vi "SHAPE_GA_Insert Into Population.vi"(6 "Parameters":T3={"Population size"=100, "Generations no."=500, "Significant digits"=4, "Crossover probabality"=0.85, "Mutation mode"=enum."one-point, fixed rate", "Use Gray code?"=FALSE, "Mutation rate"=0.05, "Min mutation rate"=0.0005, "Max mutation rate"=0.25, "Reproduction plan"=enum."Steady-state-replace-worst", "Elitism"=FALSE, "Fmax"=1} {"Max mutation rate" min=0.0 max=1.0; "Min mutation rate" min=0.0 max=1.0; "Mutation rate" min=0.0 max=1.0; "Crossover probabality" min=0.0 max=1.0; "Significant digits" min=1; "Generations no." min=1; "Population size" min=1}, 7 "Fitness Function":T2, 8 "Offsprings":i32[][](array[numeric]), 11 "Population in":T1) -> (3 "Population out":T1)   [LabVIEW 2016, in "Shapelets Search (GA).lvlib"]
doc: "Вставить потомков в популяцию с учетом стратегии замещения особей (reproduction plan)"
uses:
  Shapelets Search (GA).lvlib
  5. Features Optimization/_Optimal Frequency Bands Search/GA_core/GA_tParameters.ctl
  5. Features Optimization/_Optimal Frequency Bands Search/GA_core/GA_tFitness Function.ctl
  5. Features Optimization/_Optimal Frequency Bands Search/GA_core/GA_tPopulation.ctl
  5. Features Optimization/_Optimal Frequency Bands Search/GA_core/GeneticAlgorithm.lvlib
panel:
  # "This VI is a part of BCI Design library, http://www.ru-bci.org \nCopyright © 2020, Sotnikov Peter, All rights reserved. License: GNU GPLv3"
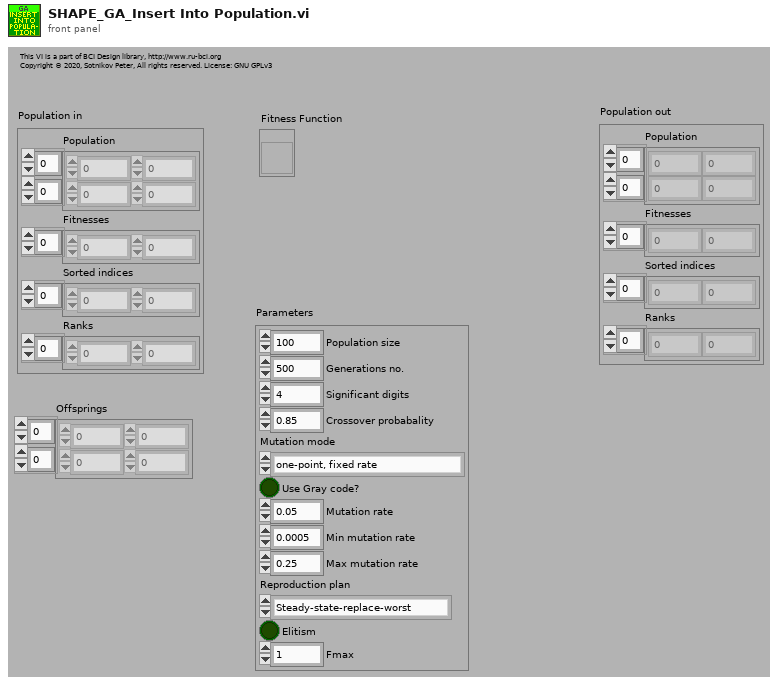
[diagram p1: front panel]
types:
  T1 = typedef "Optimal Frequency Bands Search.lvlib/GeneticAlgorithm.lvlib/GA_tPopulation.ctl" = cluster{"Population":i32[][], "Fitnesses":dbl[], "Sorted indices":i32[], "Ranks":i32[]}
  T2 = typedef "Optimal Frequency Bands Search.lvlib/GeneticAlgorithm.lvlib/GA_tFitness Function.ctl" = refnum<vi>
  T3 = typedef "Optimal Frequency Bands Search.lvlib/GeneticAlgorithm.lvlib/GA_tParameters.ctl" = cluster{"Population size":i32, "Generations no.":i32, "Significant digits":i32, "Crossover probabality":dbl, "Mutation mode":enum16{"one-point, fixed rate", "one-point, fitness-adjustable rate", "one-point, distance-adjustable rate"}, "Use Gray code?":bool, "Mutation rate":dbl, "Min mutation rate":dbl, "Max mutation rate":dbl, "Reproduction plan":enum16{"Full generational replacement", "Steady-state-replace-random", "Steady-state-replace-worst"}, "Elitism":bool, "Fmax":i32}
  T4 = enum16{"Full generational replacement", "Steady-state-replace-random", "Steady-state-replace-worst"}
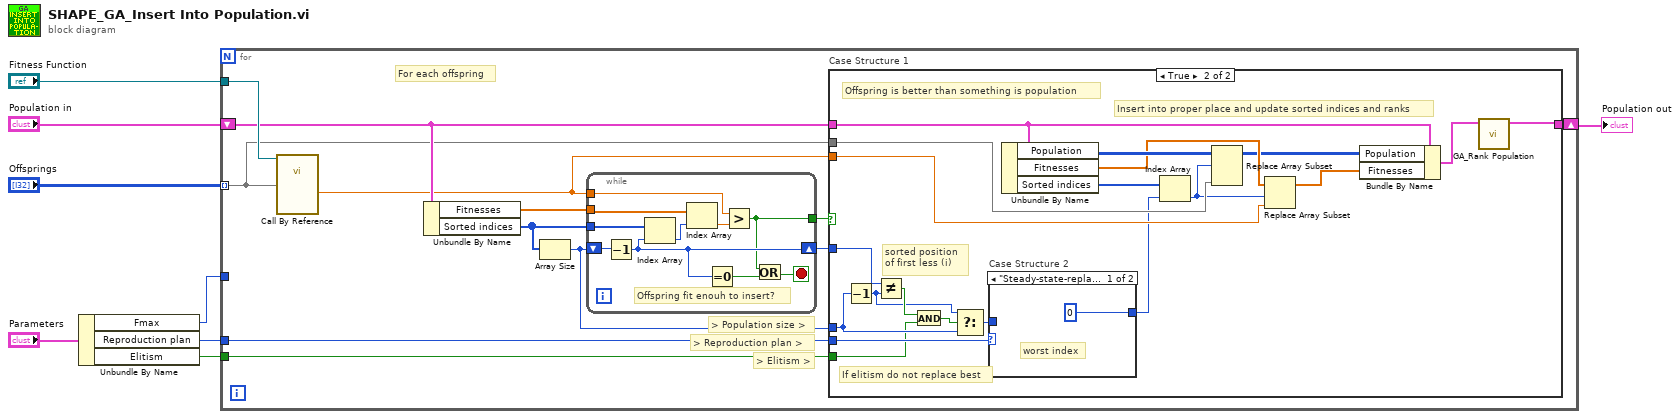
[diagram p0: block diagram]
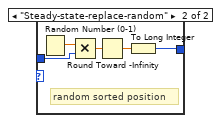
[diagram p3: hidden frame]
diagram:
  n1 = Unbundle By Name("Parameters") -> ("Fmax"=w1:i32, "Reproduction plan"=w5:T4, "Elitism"=w3:bool)
  n2 = for {
    tunnel: "Offsprings" -> [w10] mode=indexing
    shift-right: [w11] -> w2
    shift-left: "Population in" -> [w16]
    tunnel: w5 -> [w15]
    tunnel: "Fitness Function" -> [w20]
    tunnel: w3 -> [w13]
    tunnel: w1 -> [_]
    # "> Population size >"
    # "> Elitism >"
    # "> Reproduction plan >"
    # "For each offspring"
    n3 = call-by-ref "?"(reference=w20, "Phenotype"=w10) -> ("Fitness"=w9:dbl)  [unwired: 3 in, 2 out]
    n4 = Unbundle By Name(w16) -> ("Fitnesses"=w19:dbl[], "Sorted indices"=w18:i32[])
    n5 = Array Size(array=w18) -> (size(s)=w14:i32)
    n6 = while {
      tunnel: w19 -> [w55]
      tunnel: w18 -> [w56]
      shift-right: [w54] -> w12
      shift-left: w14 -> [w57]
      tunnel: w9 -> [w52]
      tunnel: [w49] -> w17
      stop <- w50 stop-if-true
      # "Offspring fit enouh to insert?"
      n7 = Decrement(x=w57) -> (x-1=w54:i32)
      n8 = Index Array(array=w56, index=w54) -> (element=w48:i32)
      n9 = Index Array(array=w55, index=w48) -> (element=w53:dbl)
      n10 = Equal To 0?(x=w54) -> (x = 0?=w51:bool)
      n11 = Greater?(x=w52, y=w53) -> (0:w49:bool)
      n12 = Or(x=w49, y=w51) -> (x .or. y?=w50:bool)
    }
    n13 = case "Case Structure 1" shown="True" w17 {
      tunnel: w16 -> [w21 w31]
      tunnel: w9 -> [_ w37]
      tunnel: w10 -> [_ w39]
      tunnel: w15 -> [_ w41]
      tunnel: w14 -> [_ w33]
      tunnel: w12 -> [_ w27]
      tunnel: w13 -> [_ w24]
      tunnel: [w21 w25] -> w11
      frame False {
        # "Offspring is worse than whole population"
      }
      frame True {
        # "Offspring is better than something is population"
        # "If elitism do not replace best"
        # "Insert into proper place and update sorted indices and ranks"
        # "sorted position \nof first less (i)"
        n14 = Decrement(x=w33) -> (x-1=w22:i32)
        n15 = Not Equal?(x=w27, y=w22) -> (x != y?=w35:bool)
        n16 = And(x=w35, y=w24) -> (x .and. y?=w34:bool)
        n17 = Select(t=w22, s=w34, f=w33) -> (s? t:f=w32:i32)
        n18 = case "Case Structure 2" shown="\"Steady-state-replace-worst\", Default" w41 {
          tunnel: w32 -> [_ w46]
          tunnel: [0 w43] -> w23
          frame "Steady-state-replace-worst", Default {
            # "worst index"
          }
          frame "Steady-state-replace-random" {
            # "random sorted position"
            n19 = Random Number (0-1)() -> (number: 0 to 1=w47:dbl)
            n20 = Multiply(x=w47, y=w46) -> (x*y=w45:dbl)
            n21 = Round Toward -Infinity(1:w45) -> (0:w44:dbl)
            n22 = To Long Integer(number=w44) -> (32bit integer=w43:i32)
          }
        }
        n23 = Unbundle By Name(w31) -> ("Population"=w40:i32[][], "Fitnesses"=w38:dbl[], "Sorted indices"=w36:i32[])
        n24 = Index Array(array=w36, index=w23) -> (element=w28:i32)
        n25 = Replace Array Subset(array=w40, new element=w39, index (row)=w28) -> (w30:i32[][])  [unwired: 1 in]
        n26 = Replace Array Subset(array=w38, new element=w37, index=w28) -> (w29:dbl[])
        n27 = Bundle By Name(cluster=w31, "Population"=w30, "Fitnesses"=w29) -> (w26:T1)
        n28 = call "GA_Rank Population.vi"("Population in"=w26) -> ("Population out"=w25:T1)  [unwired: 10 in]
      }
    }
  }
  "Population out" <- w2
